vi "Calculate DNL.vi"(8 "Error In":errorcluster, 11 "ADC in":refnum<class "ADC.lvclass">) -> (0 "Error Out":errorcluster, 1 "Monotonic?":bool, 2 "DNL Values":dbl[](array[numeric]), 3 "ADC out":refnum<class "ADC.lvclass">)   [LabVIEW 2023, in "ADC.lvclass"]
doc: "The VI calculates the DNL values for the ADC."
uses:
  ADC.lvclass
  C:/Users/Ancy.Augustin/Downloads/Tasks (2)/Tasks/Tasks/SDLC - DNL and INL Testing/SDLC - DNL and INL Testing/INL and DNL Calculation/Classes/Mode/Mode.lvclass
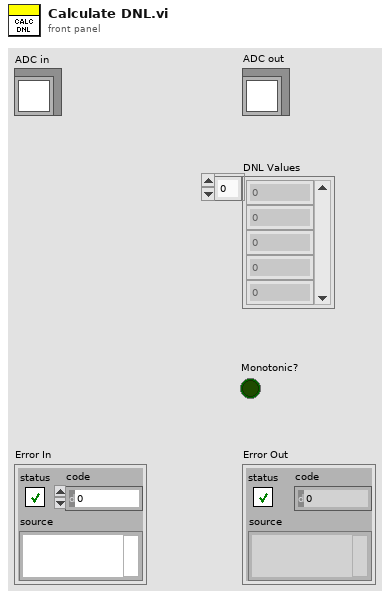
[diagram p1: front panel]
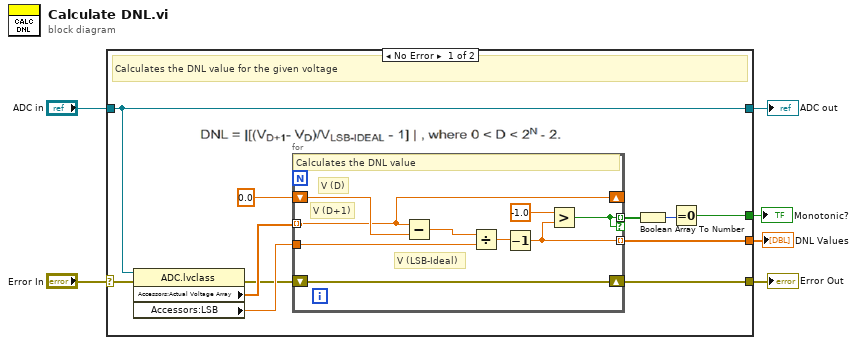
[diagram p0: block diagram]
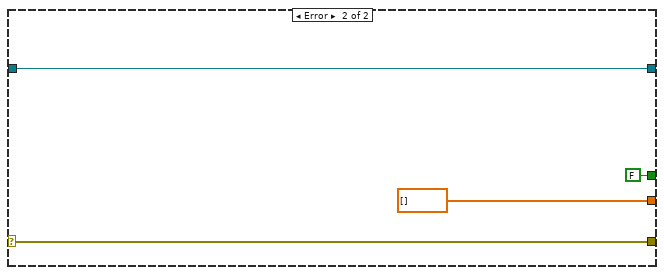
[diagram p2: hidden frame]
diagram:
  n1 = case shown="No Error" "Error In" {
    selector: "Error In" -> [w17 w30]
    tunnel: [w11 w30] -> w5
    tunnel: [w15 w29] -> w3
    tunnel: "ADC in" -> [w15 w29]
    tunnel: [w10 dbl[] []] -> w2
    tunnel: [w7 FALSE] -> w1
    frame No Error {
      # "Calculates the DNL value for the given voltage"
      n2 = property class="ADC.lvclass"(reference=w15, error in=w17) -> (error out=w12:errorcluster, "Accessors:Actual Voltage Array"=w14:dbl[], "Accessors:LSB"=w13:dbl)  [unwired: 1 out]
      n3 = for {
        tunnel: w14 -> [w22] mode=indexing
        shift-right: [w22] -> _
        shift-left: 0.0 -> [w26]
        tunnel: w13 -> [w24]
        tunnel: [w20] -> w10 mode=indexing
        shift-right: [w21] -> w11
        shift-left: w12 -> [w21]
        tunnel: [w18] -> w9 mode=indexing if=w18
        # "V (LSB-Ideal)"
        # "V (D+1)"
        # "V (D)"
        # "Calculates the DNL value"
        n4 = Subtract(x=w22, y=w26) -> (x-y=w25:dbl)
        n5 = Divide(x=w25, y=w24) -> (x/y=w23:dbl)
        n6 = Decrement(x=w23) -> (x-1=w20:dbl)
        n7 = Greater?(x=-1.0, y=w20) -> (0:w18:bool)
      }
      n8 = Boolean Array To Number(Boolean array=w9) -> (number=w8:u32)
      n9 = Equal To 0?(x=w8) -> (x = 0?=w7:bool)
    }
    frame Error {
    }
  }
  "Error Out" <- w5
  "ADC out" <- w3
  "DNL Values" <- w2
  "Monotonic?" <- w1
